vi "Delete Me.vi"() -> ()   [LabVIEW 2019, in "34980A.lvlib" / "34980A.lvclass"]
uses:
  Library/34980A.lvclass
  C:/Users/Public/Documents/Development/builds/Instruments/Instruments.lvlibp/Library/Instruments.lvclass
  Library/34980A.lvclass/34980A.ctl
  builds/Instruments/Instruments.lvlibp/Accessors/Write Resource.vi
panel:
  in  "Clear All Routes":bool
  in  "OK Button":bool
  out "MODULES":string[](array[string])
  out "error out":errorcluster
  in  "Route From":string
  in  "Route To":string
  in  "Route":bool
  in  "Send Query":bool
  in  "Send CMD":bool
  out "Response":string
  in  "command":string
  in  "stop":bool
  in  "Instrument:Config:Resource":string="TCPIP0::192.168.18.34::INSTR"
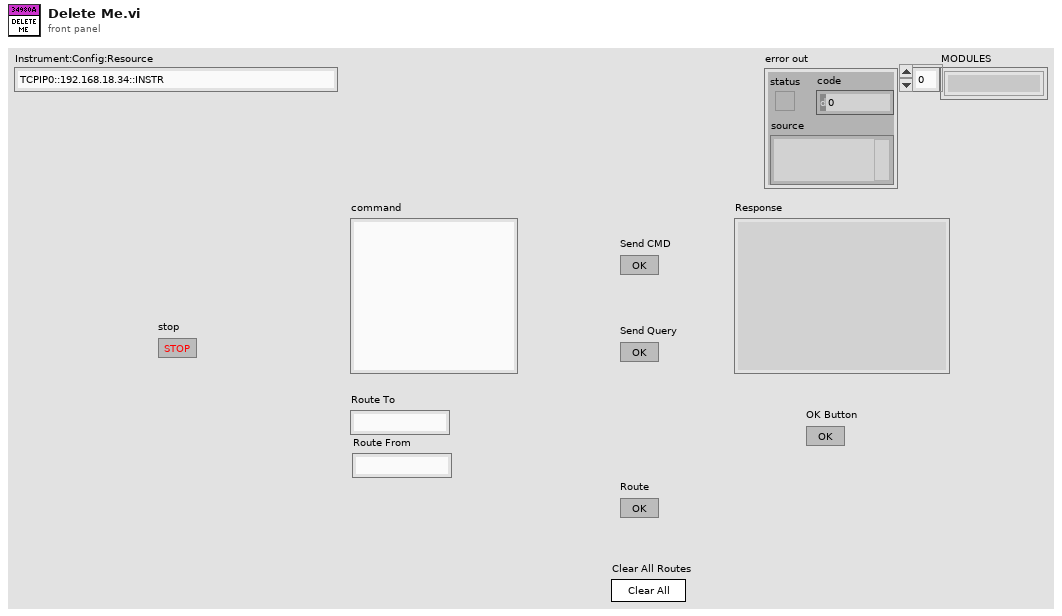
[diagram p1: front panel]
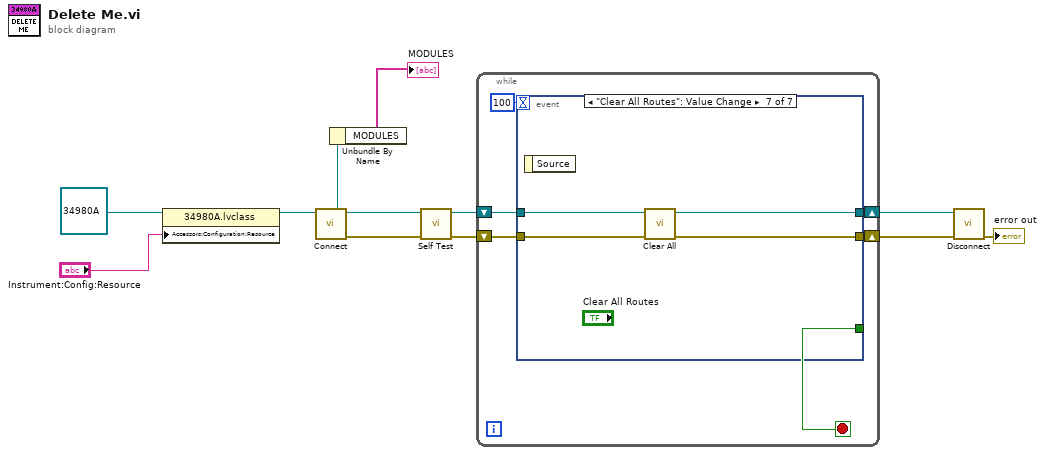
[diagram p0: block diagram]
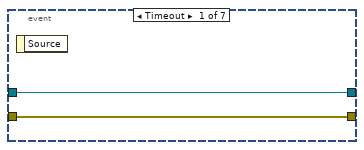
[diagram p2: hidden frame]
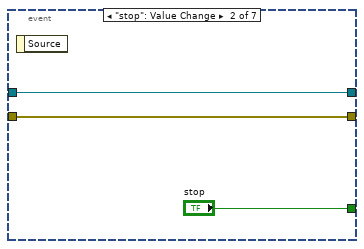
[diagram p3: hidden frame]
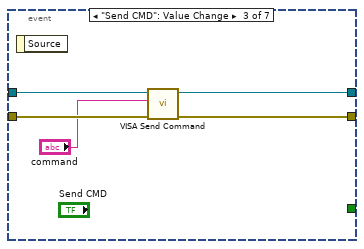
[diagram p4: hidden frame]
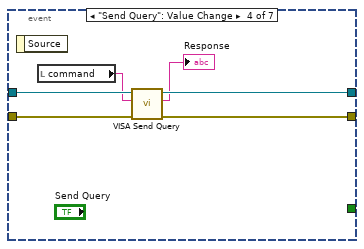
[diagram p5: hidden frame]
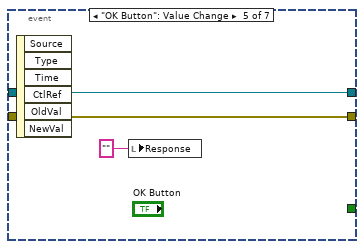
[diagram p6: hidden frame]
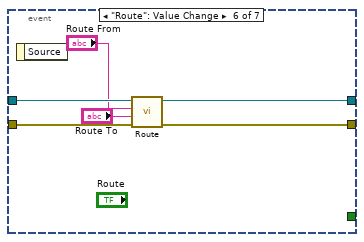
[diagram p7: hidden frame]
diagram:
  n1 = property class="34980A.lvclass"(reference=refnum<class "34980A.lvclass"> refnum ("34980A.lvlib:34980A.lvclass"), "Accessors:Configuration:Resource"="Instrument:Config:Resource") -> (reference out=w10:refnum<class "34980A.lvclass">)  [unwired: 1 in, 1 out]
  n2 = call-dynamic "Connect.vi"("34980A in"=w10) -> ("error out"=w3:errorcluster, "34980A out"=w4:refnum<class "34980A.lvclass">)  [unwired: 9 in]
  n3 = Unbundle By Name(w4) -> ("MODULES"=→"MODULES":string[])
  n4 = call-dynamic "Self Test.vi"("error in"=w3, "34980A in"=w4) -> ("error out"=w1:errorcluster, "34980A out"=w2:refnum<class "34980A.lvclass">)  [unwired: 8 in]
  n5 = while {
    shift-right: [w15] -> w8
    shift-left: w2 -> [w17]
    shift-right: [w14] -> w7
    shift-left: w1 -> [w16]
    stop <- w13 stop-if-true
    n6 = event shown="[6] \"Clear All Routes\": Value Change" {
      selector: _ -> [_ _ _ _ _ _ _]
      dyn-events: _ -> [_ _ _ _ _ _ _]
      timeout: 100 -> [_ _ _ _ _ _ _]
      tunnel: w17 -> [w19 w22 w27 w33 w36 w42 w46]
      tunnel: w16 -> [w18 w21 w26 w32 w35 w41 w45]
      tunnel: [w19 w22 w25 w30 w36 w40 w44] -> w15
      tunnel: [w18 w21 w24 w31 w35 w39 w43] -> w14
      tunnel: [_ "stop" _ _ _ _ _] -> w13
      event Timeout {
        n7 = event-data() -> ()  [unwired: 1 in, 1 out]
      }
      event "stop": Value Change {
        n8 = event-data() -> ()  [unwired: 1 in, 1 out]
      }
      event "Send CMD": Value Change {
        n9 = event-data() -> ()  [unwired: 1 in, 1 out]
        n10 = call "VISA Send Command.vi"("error in"=w26, "Command"="command", "34980A in"=w27) -> ("error out"=w24:errorcluster, "34980A out"=w25:refnum<class "34980A.lvclass">)  [unwired: 7 in]
      }
      event "Send Query": Value Change {
        n11 = event-data() -> ()  [unwired: 1 in, 1 out]
        n12 = local read "command"() -> (w29:string)
        n13 = call "VISA Send Query.vi"("error in"=w32, "Query"=w29, "34980A in"=w33) -> ("error out"=w31:errorcluster, "read buffer"=→"Response":string, "34980A out"=w30:refnum<class "34980A.lvclass">)  [unwired: 6 in]
      }
      event "OK Button": Value Change {
        n14 = event-data() -> ()  [unwired: 1 in, 6 out]
        n15 = local write "Response"("" ("Response")) -> ()
      }
      event "Route": Value Change {
        n16 = event-data() -> ()  [unwired: 1 in, 1 out]
        n17 = call "Route.vi"("error in"=w41, "Route To"="Route To", "Route From"="Route From", "34980A in"=w42) -> ("error out"=w39:errorcluster, "34980A out"=w40:refnum<class "34980A.lvclass">)  [unwired: 6 in]
      }
      event "Clear All Routes": Value Change {
        n18 = event-data() -> ()  [unwired: 1 in, 1 out]
        n19 = call-dynamic "Clear All.vi"("error in"=w45, "34980A in"=w46) -> ("error out"=w43:errorcluster, "34980A out"=w44:refnum<class "34980A.lvclass">)  [unwired: 8 in]
      }
    }
  }
  n20 = call-dynamic "Disconnect.vi"("error in"=w7, "34980A in"=w8) -> ("error out"=→"error out":errorcluster)  [unwired: 8 in, 1 out]
